vi "Reverse Direction.vi"(11 "Direction in":i32) -> (3 "Reverse Direction":i32)   [LabVIEW 2017, in "AntFarm_MB.lvclass"]
uses:
  AntFarm_MB.lvclass
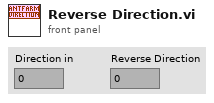
[diagram p1: front panel]
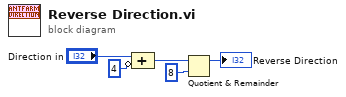
[diagram p0: block diagram]
diagram:
  n1 = Compound Arithmetic op=ADD("Direction in", invert 4 ("value")) -> (w3:i32)
  n2 = Quotient & Remainder(x=w3, y=8) -> (x-y*floor(x/y)=→"Reverse Direction":i32)  [unwired: 1 out]
